vi "Loop_HW.vi"   [LabVIEW 2017, in "Sonar.lvlib"]
uses:
  Sonar.lvlib
  <vilib>/Rock Robotics/WPI/Ultrasonic/WPI_SonarMB1010AnalogDeviceRef.ctl
  <vilib>/Rock Robotics/WPI/AnalogChannel/WPI_AnalogChannelDevRef.ctl
  <vilib>/Rock Robotics/SystemInterfaces/AI/FPGA_AIChannel.ctl
  Globals/Global_HW_Address_Assignments.vi
  Globals/Global_STOP.vi
  Global_HW_Data Out.vi
types:
  T1 = typedef "FPGA_AIChannel.ctl" = enum8{"AI 0", "AI 1", "AI 2", "AI 3", "AI MXP 0", "AI MXP 1", "AI MXP 2", "AI MXP 3", "Invalid"}
  T2 = typedef "WPI_SonarMB1010AnalogDeviceRef.ctl" = cluster{"AIDeviceRef":T3, "Scaling factor (V/in)":dbl, "Average Bits":u8}
  T3 = typedef "WPI_AnalogChannelDevRef.ctl" = cluster{"DevStatus":errorcluster, "Analog Channel":T1}
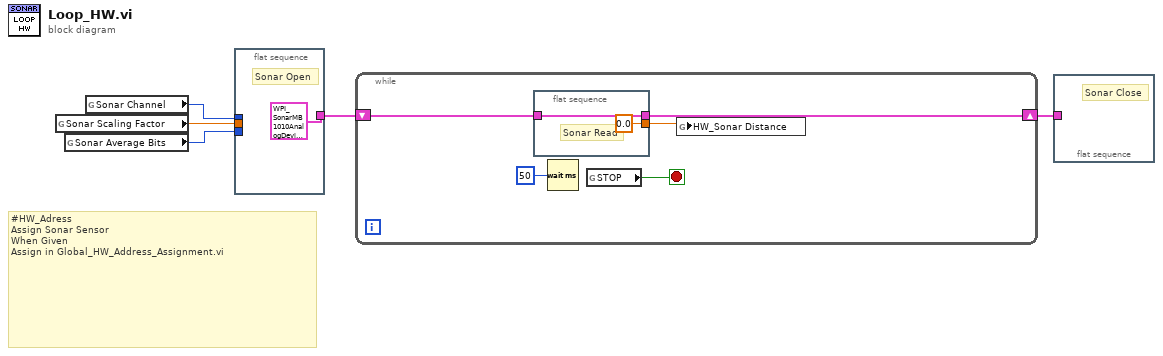
[diagram p0: block diagram]
diagram:
  # "#HW_Adress\nAssign Sonar Sensor\nWhen Given\nAssign in Global_HW_Address_Assignment.vi"
  n1 = global read "Global_HW_Address_Assignments.vi" "Sonar Scaling Factor"() -> (w2:dbl)
  n2 = global read "Global_HW_Address_Assignments.vi" "Sonar Average Bits"() -> (w1:u8)
  n3 = global read "Global_HW_Address_Assignments.vi" "Sonar Channel"() -> (w3:T1)
  n4 = flat-sequence {
    tunnel: [T2 {"AIDeviceRef"={"DevStatus"={"status"=FALSE, "code"=0, "source"=""}, "Analog Channel"=enum."Invalid"}, "Scaling factor (V/in)"=0.0098, "Average Bits"=3} ("SonarMB1010AnalogDevRef")] -> w5
    tunnel: w3 -> [_]
    tunnel: w2 -> [_]
    tunnel: w1 -> [_]
    frame #0 {
      # "Sonar Open"
    }
  }
  n5 = while {
    shift-right: [w11] -> w4
    shift-left: w5 -> [w7]
    stop <- w10 stop-if-true
    n6 = flat-sequence {
      tunnel: [w13] -> w11
      tunnel: [0.0 ("Distance")] -> w8
      tunnel: w7 -> [w13]
      frame #0 {
        # "Sonar Read"
      }
    }
    n7 = Wait (ms)(milliseconds to wait=u32 50) -> ()  [unwired: 1 out]
    n8 = global read "Global_Stop.vi" "STOP"() -> (w10:bool)
    n9 = global write "Global_HW_Data Out.vi" "HW_Sonar Distance"(w8) -> ()
  }
  n10 = flat-sequence {
    tunnel: w4 -> [_]
    frame #0 {
      # "Sonar Close"
    }
  }
